vi "loadDataIntoScript_single.vi"(8 "error in (no error)":errorcluster, 9 "Path":path=path "C:/Users/Administrator/Desktop/Crete/Lua/Sweeping/lvScript.tsp", 10 "data":dbl[][][](array[numeric]), 11 "K2602 in":refnum<class "K2602.lvclass">) -> (0 "error out":errorcluster, 2 "script":string, 3 "K2602 out":refnum<class "K2602.lvclass">)   [LabVIEW 2011, in "Hardware.lvlib" / "Channels.lvlib" / "K2602.lvclass"]
uses:
  K2602.lvclass
  K2602.lvclass/K2602.ctl
  AnalogOutput.lvclass
panel:
  out "channelConfig":string
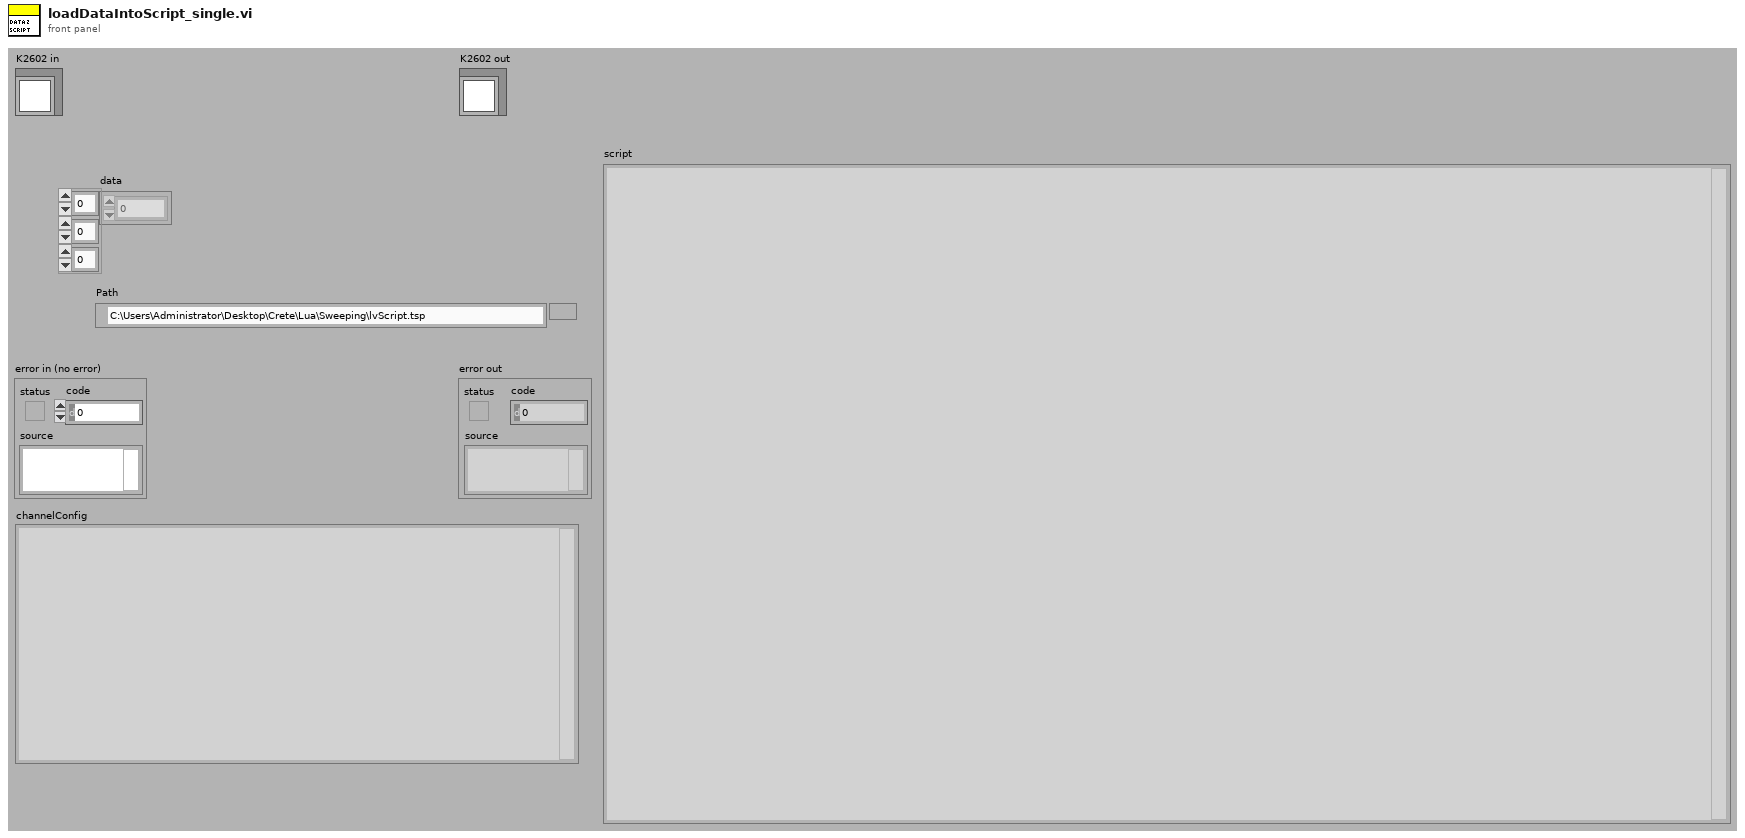
[diagram p1: front panel]
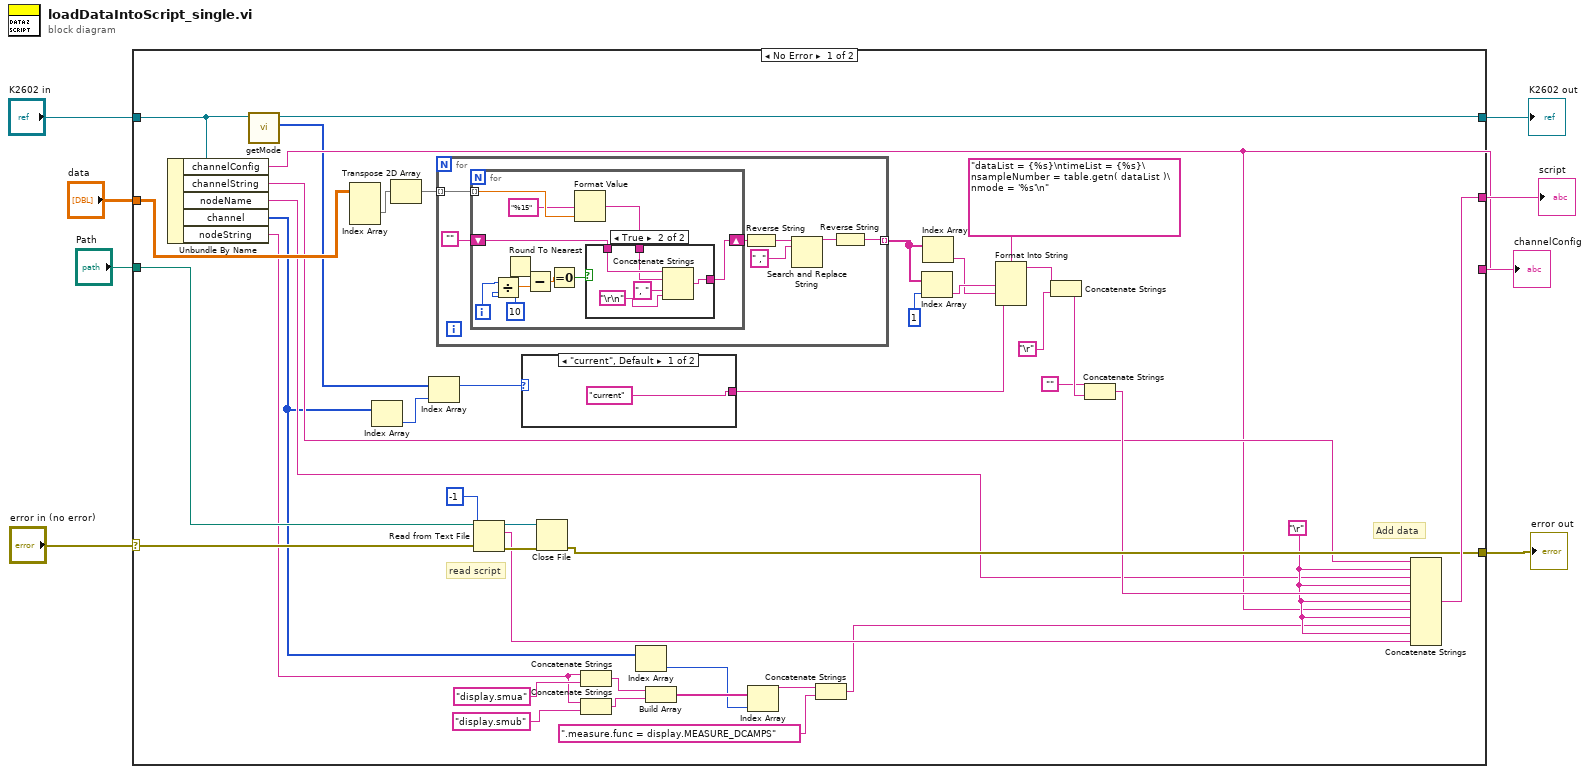
[diagram p0: block diagram]
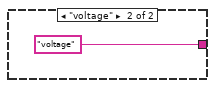
[diagram p2: hidden frame]
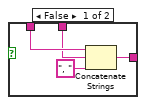
[diagram p3: hidden frame]
diagram:
  n1 = case shown="No Error" "error in (no error)" {
    selector: "error in (no error)" -> [w48 w81]
    tunnel: [w43 w81] -> w7
    tunnel: [w15 w80] -> w5
    tunnel: "K2602 in" -> [w16 w80]
    tunnel: "data" -> [w47 _]
    tunnel: "Path" -> [w50 _]
    tunnel: [w46 _] -> w2
    tunnel: [w17 _] -> w1
    frame No Error {
      w32 = "\r"
      # "Add data"
      # "read script"
      n2 = Unbundle By Name(w16) -> ("channelConfig"=w17:string, "channelString"=w21:string, "nodeName"=w20:string, "channel"=w10:i32[], "nodeString"=w18:string)
      n3 = call "getMode.vi"("AnalogOutput in"=w16) -> ("mode"=w13:enum16{"current", "voltage"}[], "AnalogOutput out"=w15:refnum<class "K2602.lvclass">)  [unwired: 8 in, 1 out]
      n4 = Index Array(array=w47) -> (element=w23:dbl[][])  [unwired: 3 in]
      n5 = Index Array(array=w10) -> (element=w11:i32)  [unwired: 1 in]
      n6 = Transpose 2D Array(2D array=w23) -> (transposed array=w25:dbl[][])
      n7 = Index Array(array=w13, index=w11) -> (element=w12:enum16{"current", "voltage"})
      n8 = for {
        tunnel: w25 -> [w59] mode=indexing
        tunnel: [w53] -> w30 mode=indexing
        n9 = for {
          tunnel: w59 -> [w70] mode=indexing
          shift-right: [w66] -> w57
          shift-left: "" -> [w68]
          i -> [w61]
          n10 = Divide(x=w61, y=10) -> (x/y=w63:dbl)
          n11 = Round To Nearest(number=w63) -> (nearest integer value=w64:dbl)
          n12 = Subtract(x=w64, y=w63) -> (x-y=w65:dbl)
          n13 = Equal To 0?(x=w65) -> (x = 0?=w62:bool)
          n14 = Format Value(format string="%15", value (0)=w70) -> (output string=w67:string)  [unwired: 1 in]
          n15 = case shown="True" w62 {
            tunnel: w68 -> [w74 w79]
            tunnel: w67 -> [w73 w78]
            tunnel: [w71 w76] -> w66
            frame False {
              n16 = Concatenate Strings(w74, w73, ", ") -> (w71:string)
            }
            frame True {
              n17 = Concatenate Strings(w79, w78, ", ", "\r\n") -> (w76:string)
            }
          }
        }
        n18 = Reverse String(1:w57) -> (0:w56:string)
        n19 = Search and Replace String(input string=w56, search string=" ,") -> (result string=w54:string)  [unwired: 6 in, 3 out]
        n20 = Reverse String(1:w54) -> (0:w53:string)
      }
      n21 = Read from Text File(file (use dialog)=w50, count=-1, error in=w48) -> (refnum out=w45:refnum<file>, text=w42:string, error out=w44:errorcluster)  [unwired: 1 in, 1 out]
      n22 = case shown="\"current\", Default" w12 {
        tunnel: ["current" "voltage"] -> w9
        frame "current", Default {
        }
        frame "voltage" {
        }
      }
      n23 = Close File(refnum=w45, error in=w44) -> (error out=w43:errorcluster)  [unwired: 1 out]
      n24 = Concatenate Strings(w18, "display.smua") -> (w38:string)
      n25 = Concatenate Strings(w18, "display.smub") -> (w37:string)
      n26 = Index Array(array=w10) -> (element=w35:i32)  [unwired: 1 in]
      n27 = Build Array(w38, w37) -> (w36:string[])
      n28 = Index Array(array=w36, index=w35) -> (element=w34:string)
      n29 = Concatenate Strings(w34, ".measure.func = display.MEASURE_DCAMPS") -> (w19:string)
      n30 = Index Array(array=w30, index=1) -> (element=w29:string)
      n31 = Index Array(array=w30) -> (element=w26:string)  [unwired: 1 in]
      n32 = Format Into String(format string="dataList = {%s}\ntimeList = {%s}\nsampleNumber = table.getn( dataList )\nmode = '%s'\n", w29, w26, w9) -> (resulting string=w27:string)  [unwired: 2 in, 1 out]
      n33 = Concatenate Strings(w27, "\r") -> (w22:string)
      n34 = Concatenate Strings("", w22) -> (w41:string)
      n35 = Concatenate Strings(w21, w32, w20, w32, w41, w32, w17, w32, w19, w32, w42) -> (w46:string)
    }
    frame Error {
    }
  }
  "error out" <- w7
  "K2602 out" <- w5
  "script" <- w2
  "channelConfig" <- w1
